vi "LongDateString2TimeStamp.vi"(10 "Cover Date":string) -> (2 "time stamp":timestamp)   [LabVIEW 2024]
uses:
  <vilib>/Utility/miscctls.llb/LVDateTimeRec.ctl
  <userlib>/_OpenG.lib/string/string.llb/openg_string.lvlib
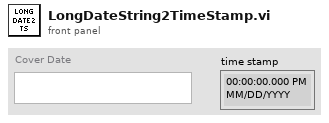
[diagram p1: front panel]
types:
  T1 = typedef "LVDateTimeRec.ctl" = cluster{"fractional second":dbl, "second":i32, "minute":i32, "hour":i32, "day of month":i32, "month":i32, "year":i32, "day of week":i32, "day of year":i32, "DST":i32}
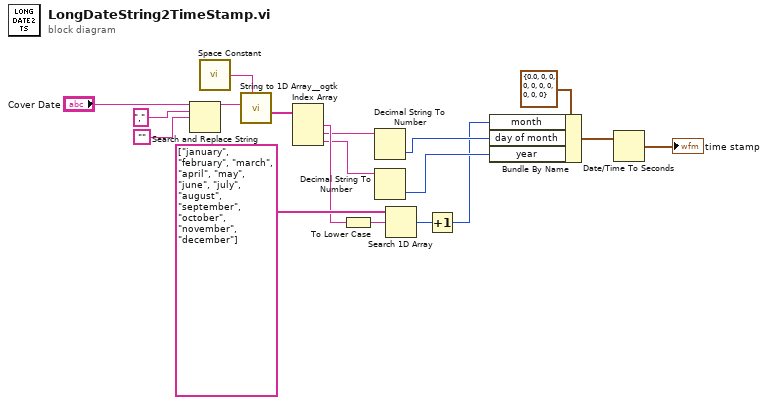
[diagram p0: block diagram]
diagram:
  n1 = Search and Replace String(input string="Cover Date", search string=",", replace string="") -> (result string=w15:string)  [unwired: 5 in, 3 out]
  n2 = call <vilib>:"Space Constant.vi"() -> ("String"=w14:string)
  n3 = call <userlib>:"String to 1D Array__ogtk.vi"("delimiter (Tab)"=w14, "string"=w15) -> ("Array of Strings"=w13:string[])  [unwired: 9 in]
  n4 = Index Array(array=w13) -> (element #1=w10:string, element #2=w7:string, element #3=w6:string)  [unwired: 3 in]
  n5 = To Lower Case(string=w10) -> (all lower case string=w12:string)
  n6 = Decimal String To Number(string=w7) -> (number=w4:i32)  [unwired: 2 in, 1 out]
  n7 = Decimal String To Number(string=w6) -> (number=w5:i32)  [unwired: 2 in, 1 out]
  n8 = Search 1D Array(1D array=string[] ["january", "february", "march", "april", "may", "june", "july", "august", "september", "october", "november", "december"], element=w12) -> (index of element=w8:i32)  [unwired: 1 in]
  n9 = Increment(x=w8) -> (x+1=w1:i32)
  n10 = Bundle By Name(cluster=T1 {"fractional second"=0.0, "second"=0, "minute"=0, "hour"=0, "day of month"=0, "month"=0, "year"=0, "day of week"=0, "day of year"=0, "DST"=0} ("date time rec"), "month"=w1, "day of month"=w4, "year"=w5) -> (w3:T1)
  n11 = Date/Time To Seconds(2:w3) -> (0:→"time stamp":timestamp)  [unwired: 1 in]
